vi "Format DescribeTagsResult_LVXML_TagSetItemType.vi"(8 "error in (no error)":errorcluster, 11 "Siblings":T3(array[cluster])) -> (0 "error out":errorcluster, 3 "Array":T1(array[cluster]))   [LabVIEW 2014, in "AWS_EC2.lvlib" / "AWS_EC2.lvclass"]
uses:
  AWS_EC2.lvclass
  lv-xml-parser/r0/trunk/VI Source/EventType.ctl
  lv-xml-parser/r0/trunk/VI Source/LV XML Parser.lvlib
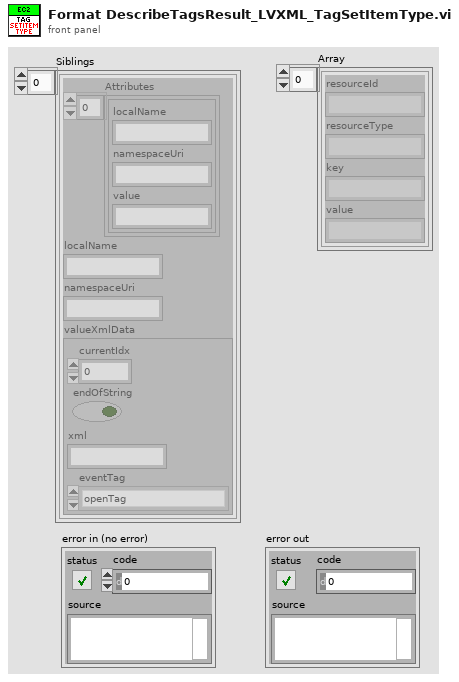
[diagram p1: front panel]
types:
  T1 = cluster{"resourceId":string, "resourceType":string, "key":string, "value":string}[]
  T2 = typedef "LV XML Parser.lvlib/EventType.ctl" = enum16{"openTag", "endOpenTag", "closeTag", "comment", "endComment", "endOfFile", "attribute", "startXml"}
  T3 = cluster{"Attributes":cluster{"localName":string, "namespaceUri":string, "value":string}[], "localName":string, "namespaceUri":string, "valueXmlData":cluster{"currentIdx":i32, "endOfString":bool, "xml":string, "eventTag":T2}}[]
  T4 = cluster{"Attributes":cluster{"localName":string, "namespaceUri":string, "value":string}[], "localName":string, "namespaceUri":string, "valueXmlData":cluster{"currentIdx":i32, "endOfString":bool, "xml":string, "eventTag":T2}}
  T5 = cluster{"currentIdx":i32, "endOfString":bool, "xml":string, "eventTag":T2}
  T6 = cluster{"namespaceUri":string, "localName":string}
  T7 = cluster{"resourceId":string, "resourceType":string, "key":string, "value":string}
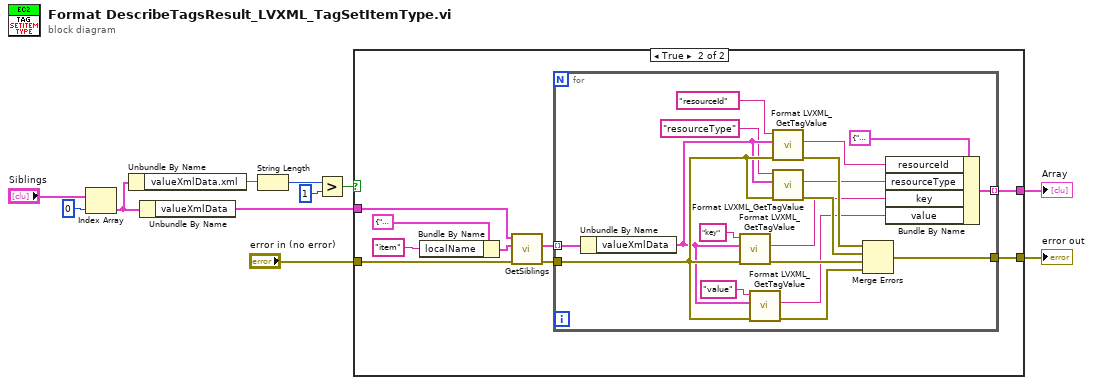
[diagram p0: block diagram]
diagram:
  n1 = Index Array(array="Siblings", index=0) -> (element=w10:T4)
  n2 = Unbundle By Name(w10) -> ("valueXmlData.xml"=w9:string)
  n3 = Unbundle By Name(w10) -> ("valueXmlData"=w8:T5)
  n4 = String Length(string=w9) -> (length=w5:i32)
  n5 = Greater?(x=w5, y=1) -> (0:w7:bool)
  n6 = case shown="True" w7 {
    tunnel: [w12 w20] -> w11
    tunnel: [_ w19] -> w1
    tunnel: "error in (no error)" -> [w12 w14]
    tunnel: w8 -> [_ w13]
    frame False {
    }
    frame True {
      n7 = Bundle By Name(cluster=T6 {"namespaceUri"="", "localName"=""} ("limitToTag"), "localName"="item" ("Tag name")) -> (w16:T6)
      n8 = call "GetSiblings.vi"("error in (no error)"=w14, "limitToTag"=w16, "xmlData"=w13) -> ("error out"=w21:errorcluster, "Siblings"=w17:T3)  [unwired: 7 in]
      n9 = for {
        tunnel: w17 -> [w39] mode=indexing
        tunnel: [w36] -> w19 mode=indexing
        tunnel: [w38] -> w20
        tunnel: w21 -> [w31]
        n10 = Unbundle By Name(w39) -> ("valueXmlData"=w30:T5)
        n11 = call "Format LVXML_GetTagValue.vi"("error in (no error)"=w31, "xmlDataIn"=w30, "Tag name"="key") -> ("error out"=w34:errorcluster, "Value"=w23:string)  [unwired: 6 in, 1 out]
        n12 = call "Format LVXML_GetTagValue.vi"("error in (no error)"=w31, "xmlDataIn"=w30, "Tag name"="value") -> ("error out"=w35:errorcluster, "Value"=w22:string)  [unwired: 6 in, 1 out]
        n13 = call "Format LVXML_GetTagValue.vi"("error in (no error)"=w31, "xmlDataIn"=w30, "Tag name"="resourceId") -> ("error out"=w32:errorcluster, "Value"=w25:string)  [unwired: 6 in, 1 out]
        n14 = call "Format LVXML_GetTagValue.vi"("error in (no error)"=w31, "xmlDataIn"=w30, "Tag name"="resourceType") -> ("error out"=w33:errorcluster, "Value"=w24:string)  [unwired: 6 in, 1 out]
        n15 = Merge Errors(w32, w33, w34, w35) -> (w38:errorcluster)
        n16 = Bundle By Name(cluster=T7 {"resourceId"="", "resourceType"="", "key"="", "value"=""} ("TagItemType"), "resourceId"=w25, "resourceType"=w24, "key"=w23, "value"=w22) -> (w36:T7)
      }
    }
  }
  "error out" <- w11
  "Array" <- w1
